vi "WriteOneSample.vi"(8 "error in (no error)":errorcluster, 11 "DaqMx_Single in":refnum<class "DaqMx_Single.lvclass">) -> (0 "error out":errorcluster, 3 "DaqMx_Single out":refnum<class "DaqMx_Single.lvclass">)   [LabVIEW 2018, in "FgenPlugins.lvlib" / "DaqMx_Single.lvclass"]
uses:
  DaqMx_Single.lvclass
  X:/Projects/PMUCal/Modules/FGen/FgenPlugins/FgenPluginBaseClass/FgenPluginsBase.lvclass
  FgenPluginBaseClass/FgenPluginsBase.lvclass/FgenPluginsBase.ctl
  MemberClasses/FunctionBaseClass/FunctionBase.lvclass/FunctionBase.ctl
  <vilib>/DAQmx/write.llb/DAQmx Write (Analog 1D Wfm NChan 1Samp).vi
  FgenPluginBaseClass/Accessors/Read FunctionClass.vi
  MemberClasses/FunctionBaseClass/Accessors/Read Waveforms.vi
  <vilib>/DAQmx/miscellaneous.llb/DAQmx Fill In Error Info.vi
  MemberClasses/FunctionBaseClass/FunctionBase.lvclass
  FgenPluginBaseClass/FgenPluginsBase.lvclass
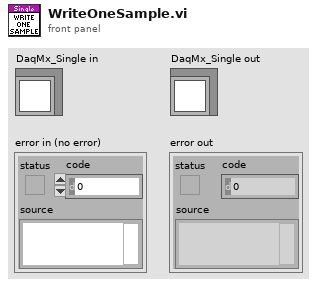
[diagram p1: front panel]
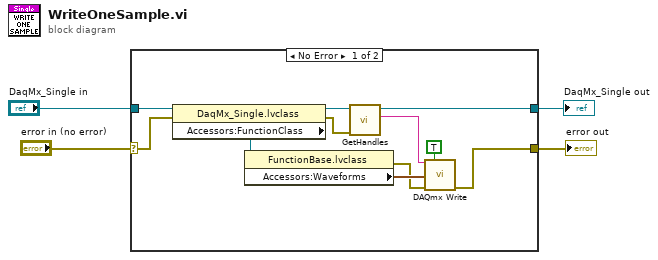
[diagram p0: block diagram]
diagram:
  n1 = case shown="No Error" "error in (no error)" {
    selector: "error in (no error)" -> [w14 w17]
    tunnel: [w10 w17] -> w3
    tunnel: [w7 w16] -> w1
    tunnel: "DaqMx_Single in" -> [w15 w16]
    frame No Error {
      n2 = property class="DaqMx_Single.lvclass"(reference=w15, error in=w14) -> (reference out=w8:refnum<class "DaqMx_Single.lvclass">, error out=w6:errorcluster, "Accessors:FunctionClass"=w13:refnum<class "FunctionBase.lvclass">)
      n3 = property class="FunctionBase.lvclass"(reference=w13) -> (error out=w11:errorcluster, "Accessors:Waveforms"=w12:waveform(dbl)[])  [unwired: 1 in, 1 out]
      n4 = call "GetHandles.vi"("error in (no error)"=w6, "FgenPluginsBase in"=w8) -> ("FirstHandle"=w5:string, "FgenPluginsBase out"=w7:refnum<class "DaqMx_Single.lvclass">)  [unwired: 6 in, 2 out]
      n5 = call-poly <vilib>:"DAQmx Write.vi"("task/channels in"=w5, "auto start"=TRUE, "data"=w12, "error in"=w11) -> ("error out"=w10:errorcluster)  [unwired: 9 in, 2 out]
    }
    frame Error {
    }
  }
  "error out" <- w3
  "DaqMx_Single out" <- w1
